vi "PubSub.vi"() -> ()   [LabVIEW 2016]
uses:
  redislib/redis-reply.ctl
  controls/MessageCluster.ctl
  controls/MessageType.ctl
panel:
  in  "Port":u16=6379
  in  "Host":string="ric700565"
  out "Events examples:":string
  out "Subscriptions Counter":i32
  in  "PUnsubscribe Button":bool
  in  "Unsubscribe Button":bool
  in  "PSubscribe Button":bool
  out "error out":errorcluster
  out "Messages":string
  in  "Channel Name":string
  in  "Subscribe Button":bool
  out "redis reply":T1
  in  "stop":bool
  # "Change before launch"
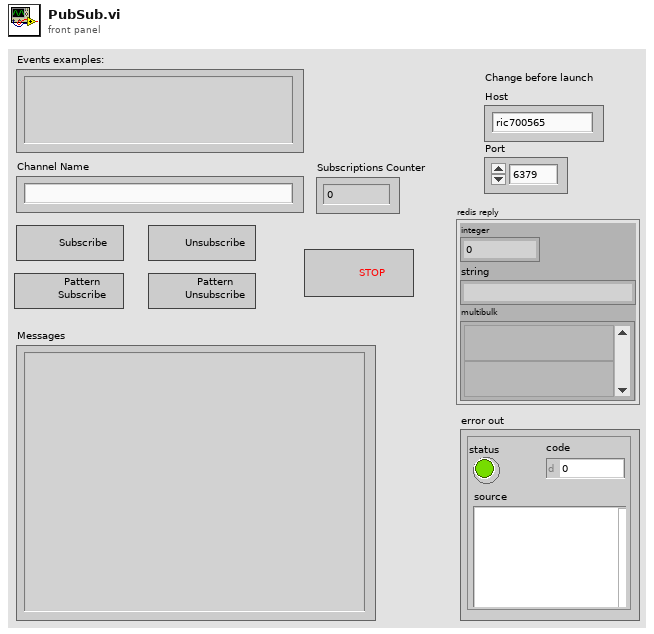
[diagram p1: front panel]
types:
  T1 = typedef "redis-reply.ctl" = cluster{"integer":i64, "string":string, "multibulk":variant[]}
  T2 = typedef "MessageCluster.ctl" = cluster{"Type":T3, "Channel":string, "Message":string, "Subscriptions":i32}
  T3 = typedef "MessageType.ctl" = enum16{"Message", "Subscribe", "Unsubscribe"}
  T4 = typedef "redis-type.ctl" = enum16{"None", "Error", "Status", "Nil", "Integer", "String", "Multibulk"}
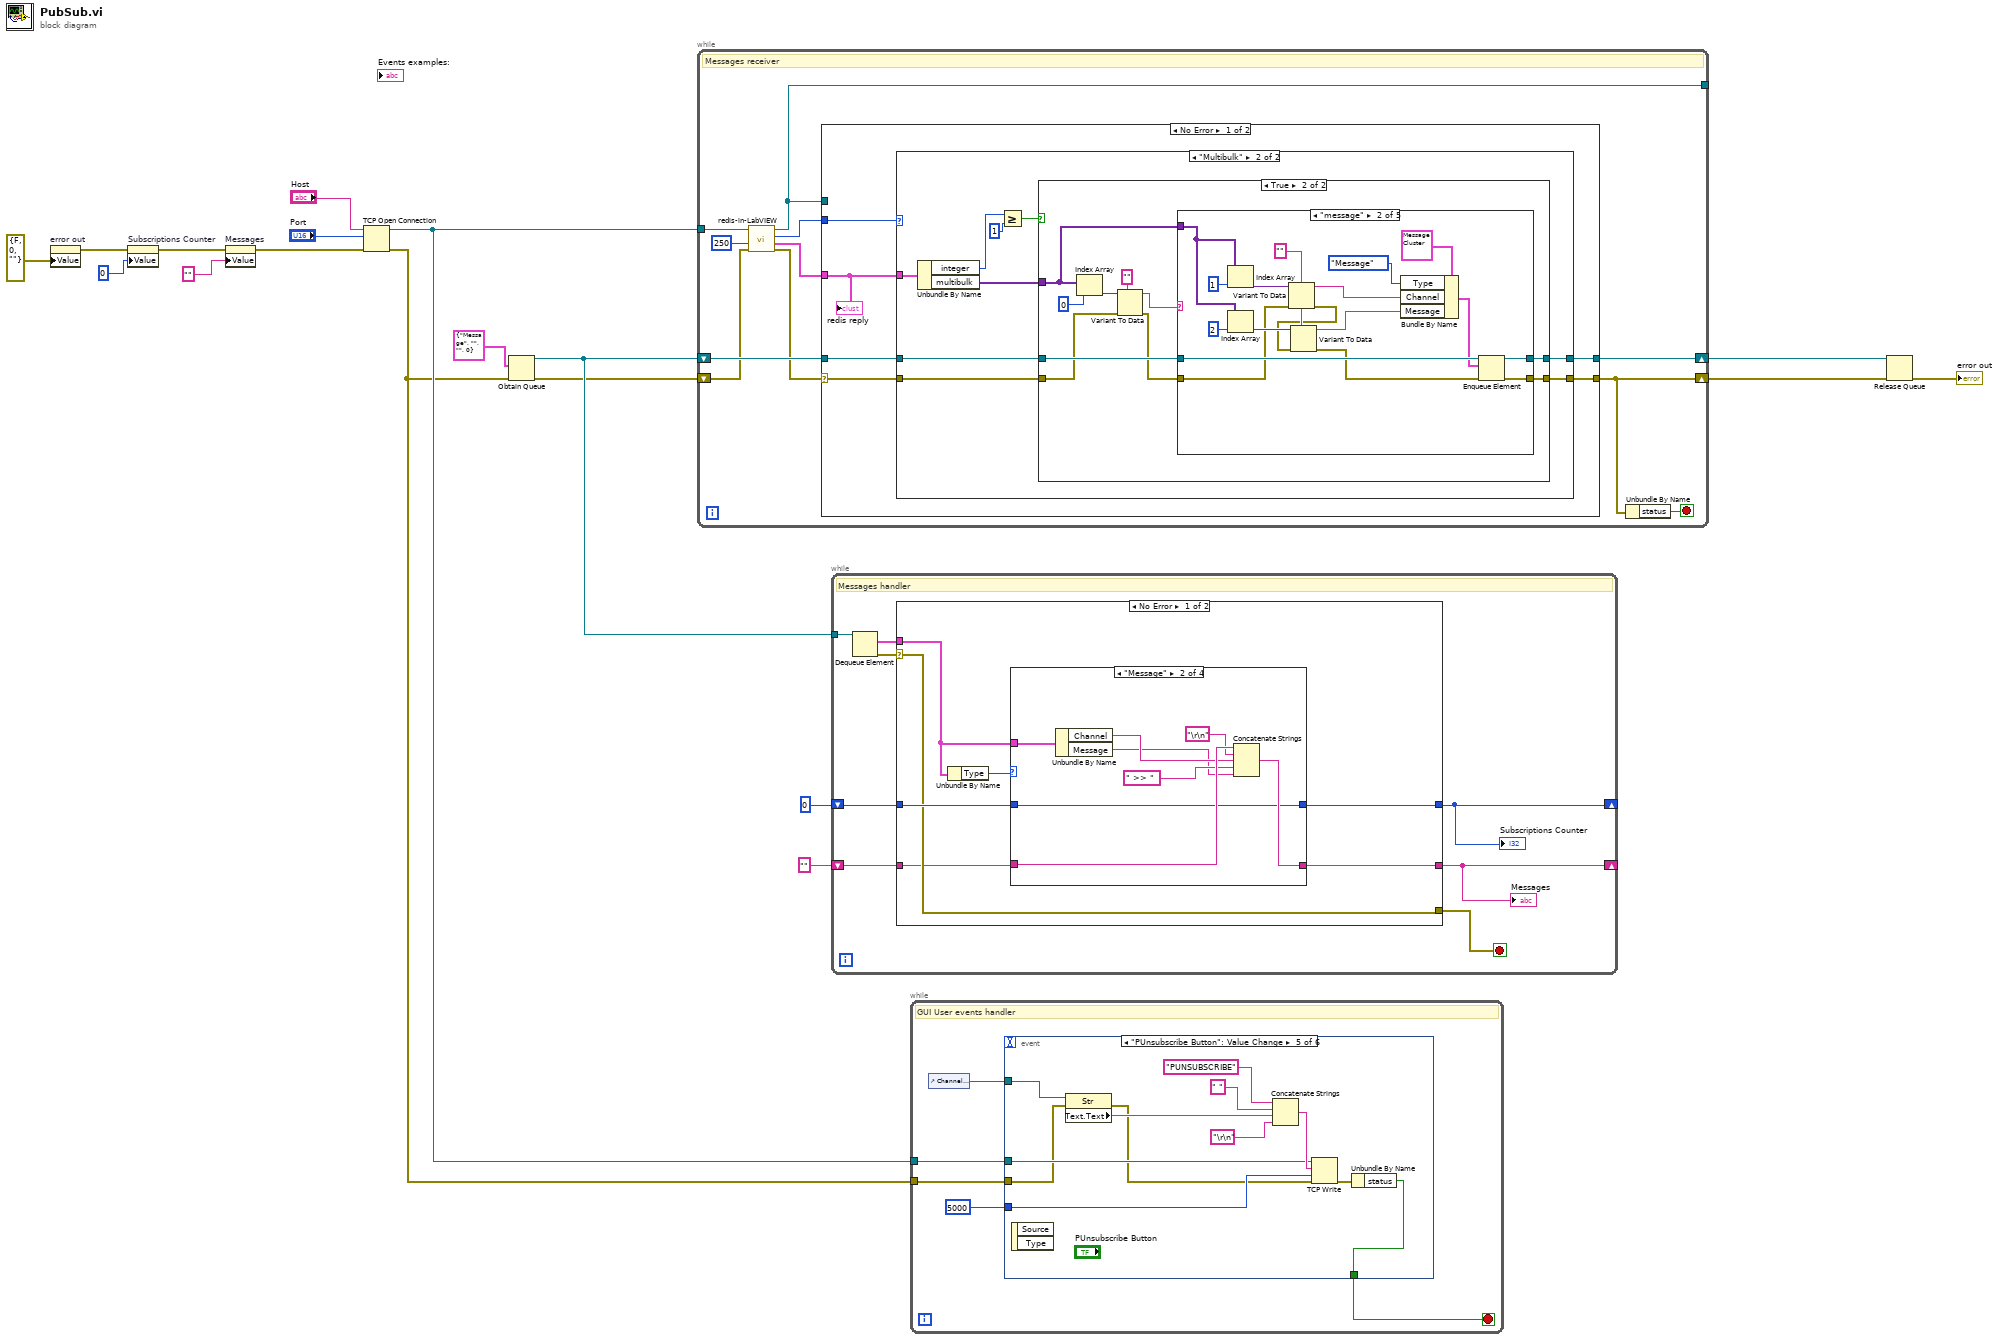
[diagram p0: block diagram]
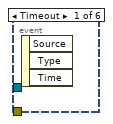
[diagram p2: hidden frame]
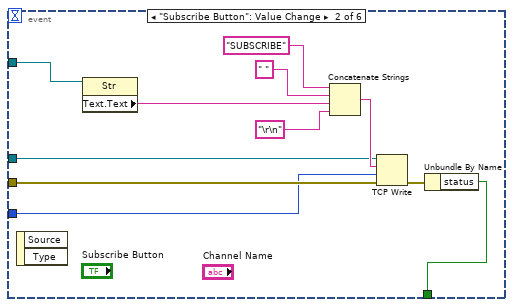
[diagram p3: hidden frame]
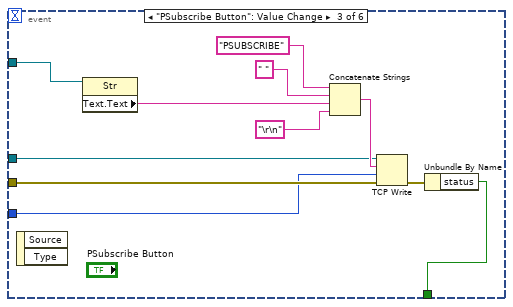
[diagram p4: hidden frame]
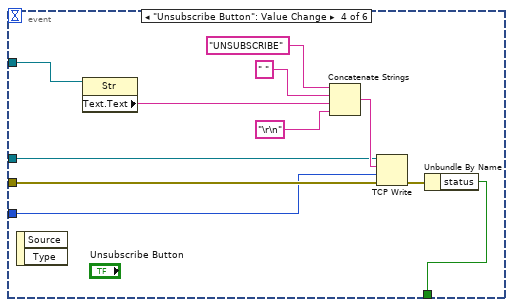
[diagram p5: hidden frame]
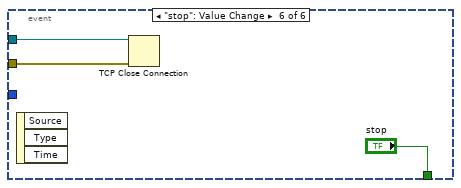
[diagram p6: hidden frame]
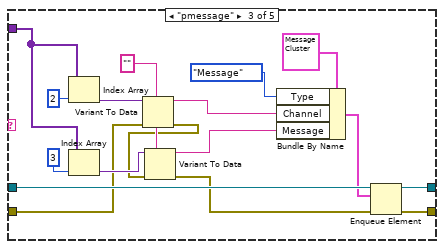
[diagram p10: hidden frame]
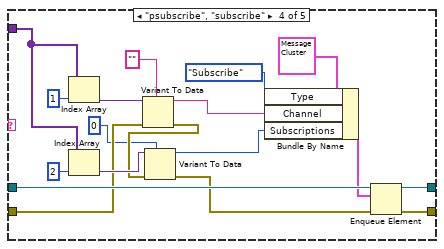
[diagram p11: hidden frame]
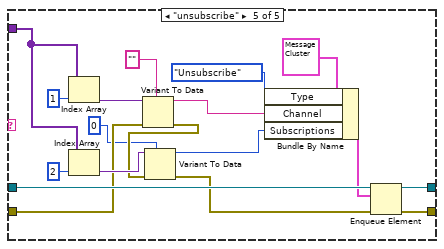
[diagram p12: hidden frame]
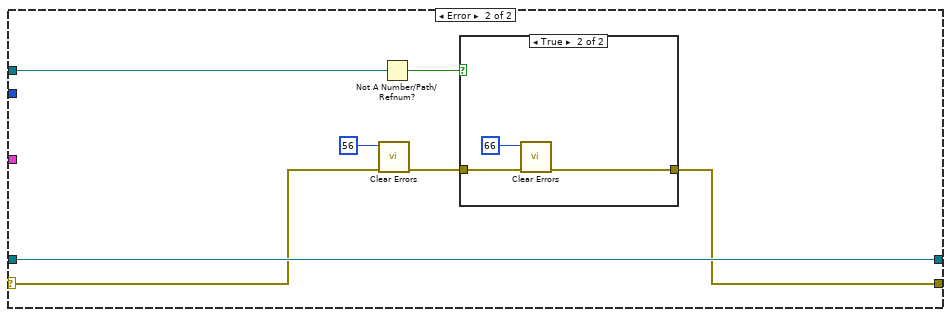
[diagram p13: hidden frame]
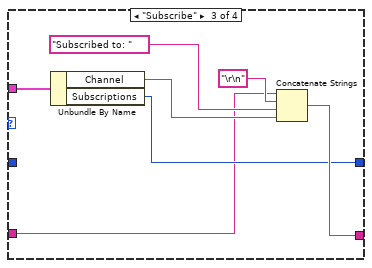
[diagram p16: hidden frame]
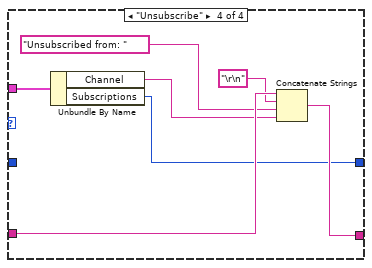
[diagram p17: hidden frame]
diagram:
  n1 = property on="error out" class="Clust (strict)"("Value"=errorcluster {"status"=FALSE, "code"=0, "source"=""} ("error constant")) -> (error out=w3:errorcluster)  [unwired: 2 in, 1 out]
  n2 = property on="Subscriptions Counter" class="DigNum (strict)"(error in=w3, "Value"=0 ("Subscriptions Counter")) -> (error out=w6:errorcluster)  [unwired: 1 in, 1 out]
  n3 = property on="Messages" class="Str"(error in=w6, "Value"="" ("Messages")) -> (error out=w7:errorcluster)  [unwired: 1 in, 1 out]
  n4 = TCP Open Connection(address="Host", remote port or service name="Port", error in (no error)=w7) -> (connection ID=w13:refnum<k5>, error out=w12:errorcluster)  [unwired: 2 in]
  n5 = Obtain Queue(element data type=T2 {"Type"=enum."Message", "Channel"="", "Message"="", "Subscriptions"=0} ("Message Cluster 3"), error in (no error)=w12) -> (queue out=w18:refnum<queue>, error out=w17:errorcluster)  [unwired: 3 in, 1 out]
  n6 = while {
    shift-right: [w21] -> w15
    shift-left: w17 -> [w26]
    shift-right: [w28] -> w16
    shift-left: w18 -> [w29]
    tunnel: w13 -> [w27]
    tunnel: [w19] -> _
    stop <- w20 stop-if-true
    # "Messages receiver"
    n7 = call "redis-in-LabVIEW.vi"("Error in"=w26, "Timeout ms"=250, "TCP in"=w27) -> ("Error out"=w24:errorcluster, "redis reply"=w23:T1, "reply type"=w22:T4, "TCP out"=w19:refnum<k5>)  [unwired: 1 in]
    n8 = case shown="No Error" w24 {
      selector: w24 -> [w32 w135]
      tunnel: w29 -> [w35 w136]
      tunnel: [w34 w136] -> w28
      tunnel: [w33 w132] -> w21
      tunnel: w23 -> [w31 _]
      tunnel: w22 -> [w30 _]
      tunnel: w19 -> [_ w134]
      frame No Error {
        n9 = case shown="\"Multibulk\"" w30 {
          tunnel: w35 -> [w37 w46]
          tunnel: [w37 w45] -> w34
          tunnel: [w36 w44] -> w33
          tunnel: w32 -> [w36 w43]
          tunnel: w31 -> [_ w42]
          frame Default {
          }
          frame "Multibulk" {
            n10 = Unbundle By Name(w42) -> ("integer"=w40:i64, "multibulk"=w41:variant[])
            n11 = Greater Or Equal?(x=w40, y=i64 1) -> (x >= y?=w38:bool)
            n12 = case shown="True" w38 {
              tunnel: w46 -> [w48 w58]
              tunnel: [w48 w57] -> w45
              tunnel: [w47 w56] -> w44
              tunnel: w43 -> [w47 w52]
              tunnel: w41 -> [_ w50]
              frame False {
              }
              frame True {
                n13 = Index Array(array=w50, index=0) -> (element=w53:variant)
                n14 = Variant To Data(error in=w52, type="" ("address"), Variant=w53) -> (data=w51:string, error out=w49:errorcluster)
                n15 = case shown="\"message\"" w51 {
                  tunnel: w58 -> [w60 w77 w94 w112 w130]
                  tunnel: [w60 w76 w93 w111 w129] -> w57
                  tunnel: w49 -> [w59 w64 w81 w100 w118]
                  tunnel: [w59 w75 w92 w110 w128] -> w56
                  tunnel: w50 -> [_ w71 w88 w106 w124]
                  frame Default {
                  }
                  frame "message" {
                    w69 = "" ("address")
                    n16 = Index Array(array=w71, index=1) -> (element=w70:variant)
                    n17 = Index Array(array=w71, index=2) -> (element=w68:variant)
                    n18 = Variant To Data(error in=w64, type=w69, Variant=w70) -> (data=w67:string, error out=w65:errorcluster)
                    n19 = Variant To Data(error in=w65, type=w69, Variant=w68) -> (data=w66:string, error out=w63:errorcluster)
                    n20 = Bundle By Name(cluster=T2 {"Type"=enum."Message", "Channel"="ch1", "Message"="ciao2", "Subscriptions"=0} ("Message Cluster 3"), "Type"=MessageType."Message", "Channel"=w67, "Message"=w66) -> (w72:T2)
                    n21 = Enqueue Element(queue=w77, element=w72, error in (no error)=w63) -> (queue out=w76:refnum<queue>, error out=w75:errorcluster)  [unwired: 1 in, 1 out]
                  }
                  frame "pmessage" {
                    w86 = "" ("address")
                    n22 = Index Array(array=w88, index=2) -> (element=w87:variant)
                    n23 = Index Array(array=w88, index=3) -> (element=w85:variant)
                    n24 = Variant To Data(error in=w81, type=w86, Variant=w87) -> (data=w84:string, error out=w82:errorcluster)
                    n25 = Variant To Data(error in=w82, type=w86, Variant=w85) -> (data=w83:string, error out=w80:errorcluster)
                    n26 = Bundle By Name(cluster=T2 {"Type"=enum."Message", "Channel"="ch1", "Message"="ciao2", "Subscriptions"=0} ("Message Cluster 3"), "Type"=MessageType."Message", "Channel"=w84, "Message"=w83) -> (w89:T2)
                    n27 = Enqueue Element(queue=w94, element=w89, error in (no error)=w80) -> (queue out=w93:refnum<queue>, error out=w92:errorcluster)  [unwired: 1 in, 1 out]
                  }
                  frame "psubscribe", "subscribe" {
                    n28 = Index Array(array=w106, index=1) -> (element=w105:variant)
                    n29 = Index Array(array=w106, index=2) -> (element=w103:variant)
                    n30 = Variant To Data(error in=w100, type="" ("address"), Variant=w105) -> (data=w102:string, error out=w101:errorcluster)
                    n31 = Variant To Data(error in=w101, type=0 ("Subscriptions"), Variant=w103) -> (data=w95:i32, error out=w99:errorcluster)
                    n32 = Bundle By Name(cluster=T2 {"Type"=enum."Message", "Channel"="ch1", "Message"="ciao2", "Subscriptions"=0} ("Message Cluster 3"), "Type"=MessageType."Subscribe", "Channel"=w102, "Subscriptions"=w95) -> (w107:T2)
                    n33 = Enqueue Element(queue=w112, element=w107, error in (no error)=w99) -> (queue out=w111:refnum<queue>, error out=w110:errorcluster)  [unwired: 1 in, 1 out]
                  }
                  frame "unsubscribe" {
                    n34 = Index Array(array=w124, index=1) -> (element=w123:variant)
                    n35 = Index Array(array=w124, index=2) -> (element=w121:variant)
                    n36 = Variant To Data(error in=w118, type="" ("address"), Variant=w123) -> (data=w120:string, error out=w119:errorcluster)
                    n37 = Variant To Data(error in=w119, type=0 ("Subscriptions"), Variant=w121) -> (data=w113:i32, error out=w117:errorcluster)
                    n38 = Bundle By Name(cluster=T2 {"Type"=enum."Message", "Channel"="ch1", "Message"="ciao2", "Subscriptions"=0} ("Message Cluster 3"), "Type"=MessageType."Unsubscribe", "Channel"=w120, "Subscriptions"=w113) -> (w125:T2)
                    n39 = Enqueue Element(queue=w130, element=w125, error in (no error)=w117) -> (queue out=w129:refnum<queue>, error out=w128:errorcluster)  [unwired: 1 in, 1 out]
                  }
                }
              }
            }
          }
        }
        "redis reply" <- w31
      }
      frame Error {
        n40 = call <vilib>:"Clear Errors.vi"("error in (no error)"=w135, "specific error code to clear (0: all)"=56) -> ("error out"=w133:errorcluster)  [unwired: 4 in, 1 out]
        n41 = Not A Number/Path/Refnum?(number/path/refnum=w134) -> (NaN/Path/Refnum?=w131:bool)
        n42 = case shown="True" w131 {
          tunnel: w133 -> [w138 w140]
          tunnel: [w138 w139] -> w132
          frame False {
          }
          frame True {
            n43 = call <vilib>:"Clear Errors.vi"("error in (no error)"=w140, "specific error code to clear (0: all)"=66) -> ("error out"=w139:errorcluster)  [unwired: 4 in, 1 out]
          }
        }
      }
    }
    n44 = Unbundle By Name(w21) -> ("status"=w20:bool)
  }
  n45 = while {
    tunnel: w18 -> [w149]
    shift-right: [w144] -> _
    shift-left: 0 ("Subscriptions") -> [w145]
    shift-right: [w143] -> _
    shift-left: "" -> [w142]
    stop <- w146 stop-if-true
    # "Messages handler"
    n46 = Dequeue Element(queue=w149) -> (element=w147:T2, error out=w148:errorcluster)  [unwired: 2 in, 2 out]
    n47 = case shown="No Error" w148 {
      selector: w148 -> [w152 w181]
      tunnel: w147 -> [w156 _]
      tunnel: [w152 w181] -> w146
      tunnel: [w154 w183] -> w144
      tunnel: w145 -> [w153 w183]
      tunnel: [w151 w182] -> w143
      tunnel: w142 -> [w150 w182]
      frame No Error {
        n48 = Unbundle By Name(w156) -> ("Type"=w155:T3)
        n49 = case shown="\"Message\"" w155 {
          tunnel: w156 -> [_ w166 w173 w180]
          tunnel: w150 -> [w158 w165 w167 w179]
          tunnel: [w158 w160 w171 w177] -> w151
          tunnel: [w157 w159 w168 w174] -> w154
          tunnel: w153 -> [w157 w159 _ _]
          frame Default {
          }
          frame "Message" {
            n50 = Unbundle By Name(w166) -> ("Channel"=w163:string, "Message"=w161:string)
            n51 = Concatenate Strings(w165, "\r\n" ("data in"), w163, " >> " ("string"), w161) -> (w160:string)
          }
          frame "Subscribe" {
            n52 = Unbundle By Name(w173) -> ("Channel"=w169:string, "Subscriptions"=w168:i32)
            n53 = Concatenate Strings(w167, "\r\n" ("data in"), "Subscribed to: " ("data in"), w169) -> (w171:string)
          }
          frame "Unsubscribe" {
            n54 = Unbundle By Name(w180) -> ("Channel"=w175:string, "Subscriptions"=w174:i32)
            n55 = Concatenate Strings(w179, "\r\n" ("data in"), "Unsubscribed from: " ("data in"), w175) -> (w177:string)
          }
        }
      }
      frame Error {
      }
    }
    "Messages" <- w143
    "Subscriptions Counter" <- w144
  }
  n56 = while {
    tunnel: w13 -> [w188]
    tunnel: w12 -> [w187]
    stop <- w186 stop-if-true
    # "GUI User events handler"
    n57 = control-ref of="Channel Name"() -> (w184:refnum<vi>)
    n58 = event shown="[4] \"PUnsubscribe Button\": Value Change" {
      selector: _ -> [_ _ _ _ _ _]
      dyn-events: _ -> [_ _ _ _ _ _]
      timeout: _ -> [_ _ _ _ _ _]
      tunnel: w188 -> [_ w195 w206 w217 w229 w235]
      tunnel: w187 -> [_ w194 w205 w216 w224 w234]
      tunnel: [_ w191 w202 w213 w226 "stop"] -> w186
      tunnel: 5000 ("timeout ms (25000)") -> [_ w193 w204 w215 w228 _]
      tunnel: w184 -> [_ w190 w201 w212 w222 _]
      event Timeout {
        n59 = event-data() -> ()  [unwired: 1 in, 3 out]
      }
      event "Subscribe Button": Value Change {
        n60 = event-data() -> ()  [unwired: 1 in, 2 out]
        n61 = property on="Property Node" class="Str"(reference=w190) -> ("Text.Text"=w189:string)  [unwired: 1 in, 2 out]
        n62 = Concatenate Strings("SUBSCRIBE" ("Command"), " " ("data in"), w189, "\r\n" ("data in")) -> (w198:string)
        n63 = TCP Write(connection ID=w195, data in=w198, error in (no error)=w194, 9:w193) -> (error out=w192:errorcluster)  [unwired: 2 out]
        n64 = Unbundle By Name(w192) -> ("status"=w191:bool)
      }
      event "PSubscribe Button": Value Change {
        n65 = event-data() -> ()  [unwired: 1 in, 2 out]
        n66 = property on="Property Node" class="Str"(reference=w201) -> ("Text.Text"=w200:string)  [unwired: 1 in, 2 out]
        n67 = Concatenate Strings("PSUBSCRIBE" ("Command"), " " ("data in"), w200, "\r\n" ("data in")) -> (w209:string)
        n68 = TCP Write(connection ID=w206, data in=w209, error in (no error)=w205, 9:w204) -> (error out=w203:errorcluster)  [unwired: 2 out]
        n69 = Unbundle By Name(w203) -> ("status"=w202:bool)
      }
      event "Unsubscribe Button": Value Change {
        n70 = event-data() -> ()  [unwired: 1 in, 2 out]
        n71 = property on="Property Node" class="Str"(reference=w212) -> ("Text.Text"=w211:string)  [unwired: 1 in, 2 out]
        n72 = Concatenate Strings("UNSUBSCRIBE" ("Command"), " " ("data in"), w211, "\r\n" ("data in")) -> (w220:string)
        n73 = TCP Write(connection ID=w217, data in=w220, error in (no error)=w216, 9:w215) -> (error out=w214:errorcluster)  [unwired: 2 out]
        n74 = Unbundle By Name(w214) -> ("status"=w213:bool)
      }
      event "PUnsubscribe Button": Value Change {
        n75 = event-data() -> ()  [unwired: 1 in, 2 out]
        n76 = property on="Property Node" class="Str"(reference=w222, error in=w224) -> (error out=w223:errorcluster, "Text.Text"=w225:string)  [unwired: 1 out]
        n77 = Concatenate Strings("PUNSUBSCRIBE" ("Command"), " " ("data in"), w225, "\r\n" ("data in")) -> (w232:string)
        n78 = TCP Write(connection ID=w229, data in=w232, error in (no error)=w223, 9:w228) -> (error out=w227:errorcluster)  [unwired: 2 out]
        n79 = Unbundle By Name(w227) -> ("status"=w226:bool)
      }
      event "stop": Value Change {
        n80 = event-data() -> ()  [unwired: 1 in, 3 out]
        n81 = TCP Close Connection(connection ID=w235, error in (no error)=w234) -> ()  [unwired: 1 in, 2 out]
      }
    }
  }
  n82 = Release Queue(queue=w16, error in (no error)=w15) -> (error out=→"error out":errorcluster)  [unwired: 1 in, 2 out]
